vi "MSEditor_WriteMethodIntoRT.vi"(8 "error in":errorcluster, 10 "Mthd in":T1, 11 "listbox ref in":refnum<vi>) -> (0 "error out":errorcluster, 3 "listbox ref out":refnum<vi>)   [LabVIEW 2018]
uses:
  Ctl/WfmCmd_Type.ctl
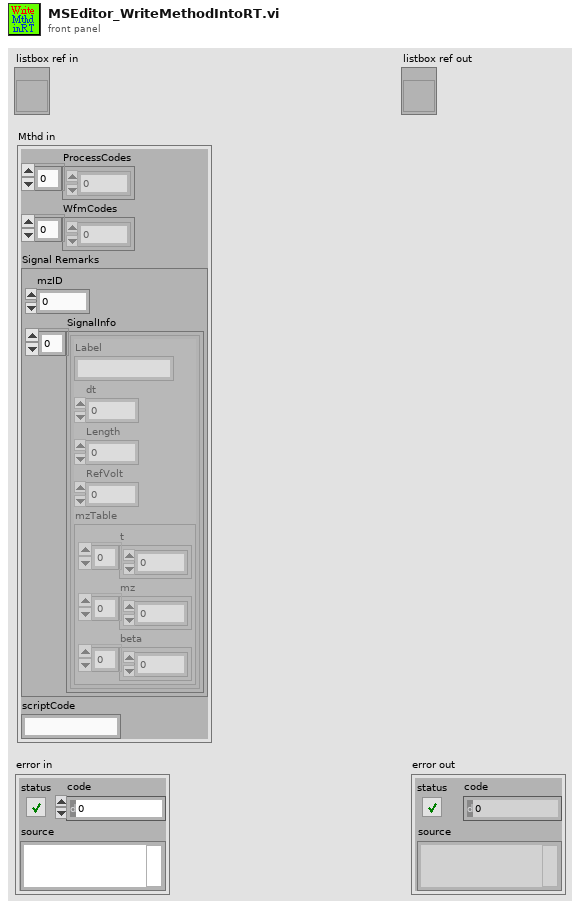
[diagram p1: front panel]
types:
  T1 = cluster{"ProcessCodes":u64[], "WfmCodes":u64[], "Signal Remarks":cluster{"mzID":u64, "SignalInfo":cluster{"Label":string, "dt":dbl, "Length":u32, "RefVolt":dbl, "mzTable":cluster{"t":dbl[], "mz":dbl[], "beta":dbl[]}}[]}, "scriptCode":string}
  T2 = typedef "WfmCmd_Type.ctl" = enum8{"None", "WFM", "EventCodes"}
  T3 = cluster{"mzID":u64, "SignalInfo":cluster{"Label":string, "dt":dbl, "Length":u32, "RefVolt":dbl, "mzTable":cluster{"t":dbl[], "mz":dbl[], "beta":dbl[]}}[]}
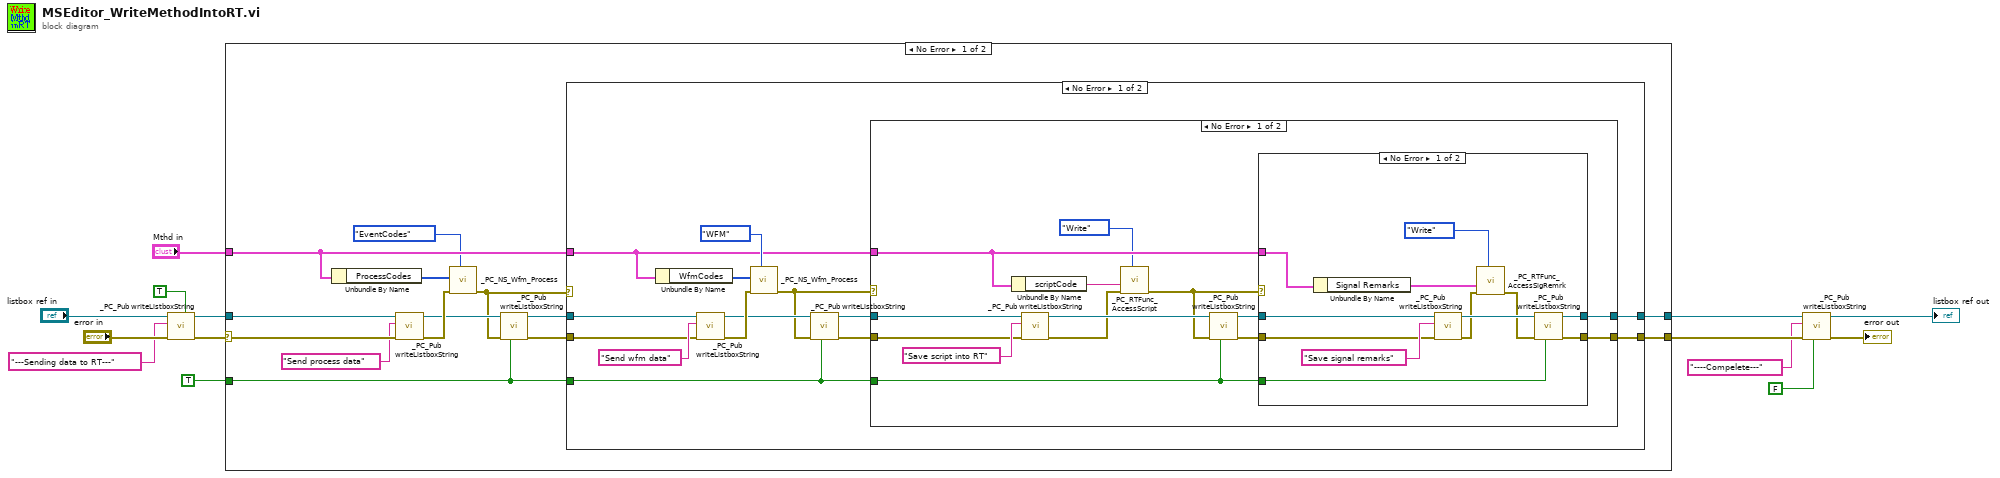
[diagram p0: block diagram]
diagram:
  n1 = call "_PC_Pub writeListboxString.vi"("Reset (F)"=TRUE, "error in (no error)"="error in", "update_Str"="---Sending data to RT---" ("New string"), "Listbox Ref Input"="listbox ref in") -> ("error out"=w10:errorcluster, "Listbox Ref Output"=w11:refnum<vi>)  [unwired: 6 in]
  n2 = case shown="No Error" w10 {
    selector: w10 -> [w22 w76]
    tunnel: "Mthd in" -> [w26 _]
    tunnel: [w28 w76] -> w12
    tunnel: w11 -> [w25 w75]
    tunnel: TRUE ("Display Error Msg? (T)") -> [w24 _]
    tunnel: [w23 w75] -> w13
    frame No Error {
      n3 = Unbundle By Name(w26) -> ("ProcessCodes"=w27:u64[])
      n4 = call "_PC_Pub writeListboxString.vi"("error in (no error)"=w22, "update_Str"="Send process data" ("New string"), "Listbox Ref Input"=w25) -> ("error out"=w20:errorcluster, "Listbox Ref Output"=w18:refnum<vi>)  [unwired: 7 in]
      n5 = call "_PC_NS_Wfm_Process.vi"("Wfm_Type"=WfmCmd_Type."EventCodes", "error in (no error)"=w20, "WfmData_U64 in"=w27) -> ("error out"=w16:errorcluster)  [unwired: 8 in]
      n6 = call "_PC_Pub writeListboxString.vi"("Display Error Msg? (F)"=w24, "error in (no error)"=w16, "Listbox Ref Input"=w18) -> ("error out"=w15:errorcluster, "Listbox Ref Output"=w17:refnum<vi>)  [unwired: 7 in]
      n7 = case shown="No Error" w16 {
        tunnel: w26 -> [w39 _]
        tunnel: [w42 w73] -> w28
        tunnel: w24 -> [w36 _]
        tunnel: w17 -> [w35 w74]
        tunnel: [w32 w74] -> w23
        tunnel: w15 -> [w29 w73]
        frame No Error {
          n8 = Unbundle By Name(w39) -> ("WfmCodes"=w40:u64[])
          n9 = call "_PC_Pub writeListboxString.vi"("error in (no error)"=w29, "update_Str"="Send wfm data" ("New string"), "Listbox Ref Input"=w35) -> ("error out"=w38:errorcluster, "Listbox Ref Output"=w34:refnum<vi>)  [unwired: 7 in]
          n10 = call "_PC_NS_Wfm_Process.vi"("Wfm_Type"=WfmCmd_Type."WFM", "error in (no error)"=w38, "WfmData_U64 in"=w40) -> ("error out"=w30:errorcluster)  [unwired: 8 in]
          n11 = call "_PC_Pub writeListboxString.vi"("Display Error Msg? (F)"=w36, "error in (no error)"=w30, "Listbox Ref Input"=w34) -> ("error out"=w31:errorcluster, "Listbox Ref Output"=w33:refnum<vi>)  [unwired: 7 in]
          n12 = case shown="No Error" w30 {
            tunnel: w39 -> [w47 _]
            tunnel: [w56 w71] -> w42
            tunnel: w36 -> [w54 _]
            tunnel: w33 -> [w53 w72]
            tunnel: [w50 w72] -> w32
            tunnel: w31 -> [w48 w71]
            frame No Error {
              n13 = Unbundle By Name(w47) -> ("scriptCode"=w45:string)
              n14 = call "_PC_Pub writeListboxString.vi"("error in (no error)"=w48, "update_Str"="Save script into RT" ("New string"), "Listbox Ref Input"=w53) -> ("error out"=w43:errorcluster, "Listbox Ref Output"=w52:refnum<vi>)  [unwired: 7 in]
              n15 = call "_PC_RTFunc_AccessScript.vi"("Function"=enum16{"Write", "Read"}."Write", "error in (no error)"=w43, "Var in"=w45) -> ("error out"=w46:errorcluster)  [unwired: 7 in, 1 out]
              n16 = call "_PC_Pub writeListboxString.vi"("Display Error Msg? (F)"=w54, "error in (no error)"=w46, "Listbox Ref Input"=w52) -> ("error out"=w49:errorcluster, "Listbox Ref Output"=w51:refnum<vi>)  [unwired: 7 in]
              n17 = case shown="No Error" w46 {
                tunnel: w47 -> [w62 _]
                tunnel: [w61 w69] -> w56
                tunnel: w54 -> [w67 _]
                tunnel: w51 -> [w65 w70]
                tunnel: [w64 w70] -> w50
                tunnel: w49 -> [w63 w69]
                frame No Error {
                  n18 = Unbundle By Name(w62) -> ("Signal Remarks"=w58:T3)
                  n19 = call "_PC_Pub writeListboxString.vi"("error in (no error)"=w63, "update_Str"="Save signal remarks" ("New string"), "Listbox Ref Input"=w65) -> ("error out"=w60:errorcluster, "Listbox Ref Output"=w66:refnum<vi>)  [unwired: 7 in]
                  n20 = call "_PC_RTFunc_AccessSigRemrk.vi"("Function"=enum16{"Write", "Read"}."Write", "error in (no error)"=w60, "Var in"=w58) -> ("error out"=w59:errorcluster)  [unwired: 7 in, 1 out]
                  n21 = call "_PC_Pub writeListboxString.vi"("Display Error Msg? (F)"=w67, "error in (no error)"=w59, "Listbox Ref Input"=w66) -> ("error out"=w61:errorcluster, "Listbox Ref Output"=w64:refnum<vi>)  [unwired: 7 in]
                }
                frame Error {
                }
              }
            }
            frame Error {
            }
          }
        }
        frame Error {
        }
      }
    }
    frame Error {
    }
  }
  n22 = call "_PC_Pub writeListboxString.vi"("Display Error Msg? (F)"=FALSE ("Display Error Msg? (T)"), "error in (no error)"=w12, "update_Str"="----Compelete---" ("New string"), "Listbox Ref Input"=w13) -> ("error out"=→"error out":errorcluster, "Listbox Ref Output"=→"listbox ref out":refnum<vi>)  [unwired: 6 in]
